vi "Create Measurement Client.vi"() -> ()   [LabVIEW 2021, in "Measurement Client.lvlib"]
uses:
  Measurement Client Utility/Measurement Client.lvlib
  Queue Driver/controls/Queue Operations.ctl
  Measurement Client Utility/subVIs/Data Holder.ctl
  <vilib>/gRPC/LabVIEW gRPC Library/Shared/grpcId.ctl
  <vilib>/Utility/miscctls.llb/LVPoint32TypeDef.ctl
  <vilib>/gRPC/Generated APIs/ni/measurementlink/discovery/v1/RPC Messages/ni_measurementlink_discovery_v1_EnumerateServicesRequest.ctl
  <vilib>/Utility/error.llb/DialogType.ctl
  <vilib>/gRPC/Generated APIs/ni/measurementlink/discovery/v1/ni.measurementlink.discovery.v1.api.lvlib
  <vilib>/Plug-In SDKs/Clients/Discovery V1/NI Discovery V1 Client.lvlib
  <vilib>/gRPC/LabVIEW gRPC Library/grpc-lvsupport-release.lvlib
panel:
  in  "Select All":bool
  in  "Next":bool
  in  "Refresh":bool
  in  "Available Measurements":i32(listbox)
  out "Active Project Name":string
  # "* Project in which the measurement client vi will be created"
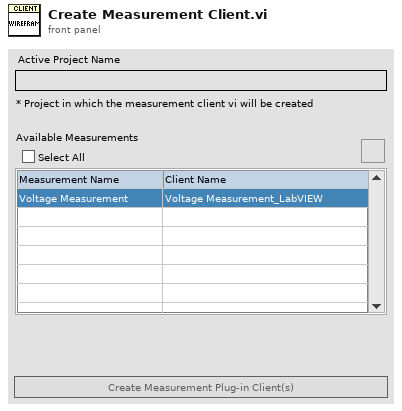
[diagram p1: front panel]
types:
  T1 = typedef "Queue Operations.ctl" = enum16{"Create Q", "Enqueue", "Enqueue N", "Dequeue", "Flush", "Release"}
  T2 = typedef "Measurement Client.lvlib/Data Holder.ctl" = cluster{"gRPCid":T3, "Services":string[][], "MosueDown Coords":T4, "No of Meas":i32, "Select All?":bool}
  T3 = typedef "grpc-lvsupport-release.lvlib/grpcId.ctl" = u64
  T4 = typedef "LVPoint32TypeDef.ctl" = cluster{"Horizontal":i32, "Vertical":i32}
  T5 = enum8{"Enabled", "Disabled", "Disabled and Grayed Out"}
  T6 = typedef "ni.measurementlink.discovery.v1.api.lvlib/ni_measurementlink_discovery_v1_EnumerateServicesRequest.ctl" = cluster{"provided_interface":string}
  T7 = typedef "LVRowAndColumnTypeDef.ctl" = cluster{"Row":i32, "Column":i32}
  T8 = typedef "ni.measurementlink.discovery.v1.api.lvlib/ni_measurementlink_discovery_v1_EnumerateServicesResponse.ctl" = cluster{"available_services":T9[]}
  T9 = typedef "ni.measurementlink.discovery.v1.api.lvlib/ni_measurementlink_discovery_v1_ServiceDescriptor.ctl" = cluster{"display_name":string, "description_url":string, "provided_interfaces":string[], "service_class":string, "annotations":T10[]}
  T10 = typedef "ni.measurementlink.discovery.v1.api.lvlib/ni_measurementlink_discovery_v1_ServiceDescriptor_AnnotationsEntry.ctl" = cluster{"key":string, "value":string}
  T11 = typedef "DialogType.ctl" = u16
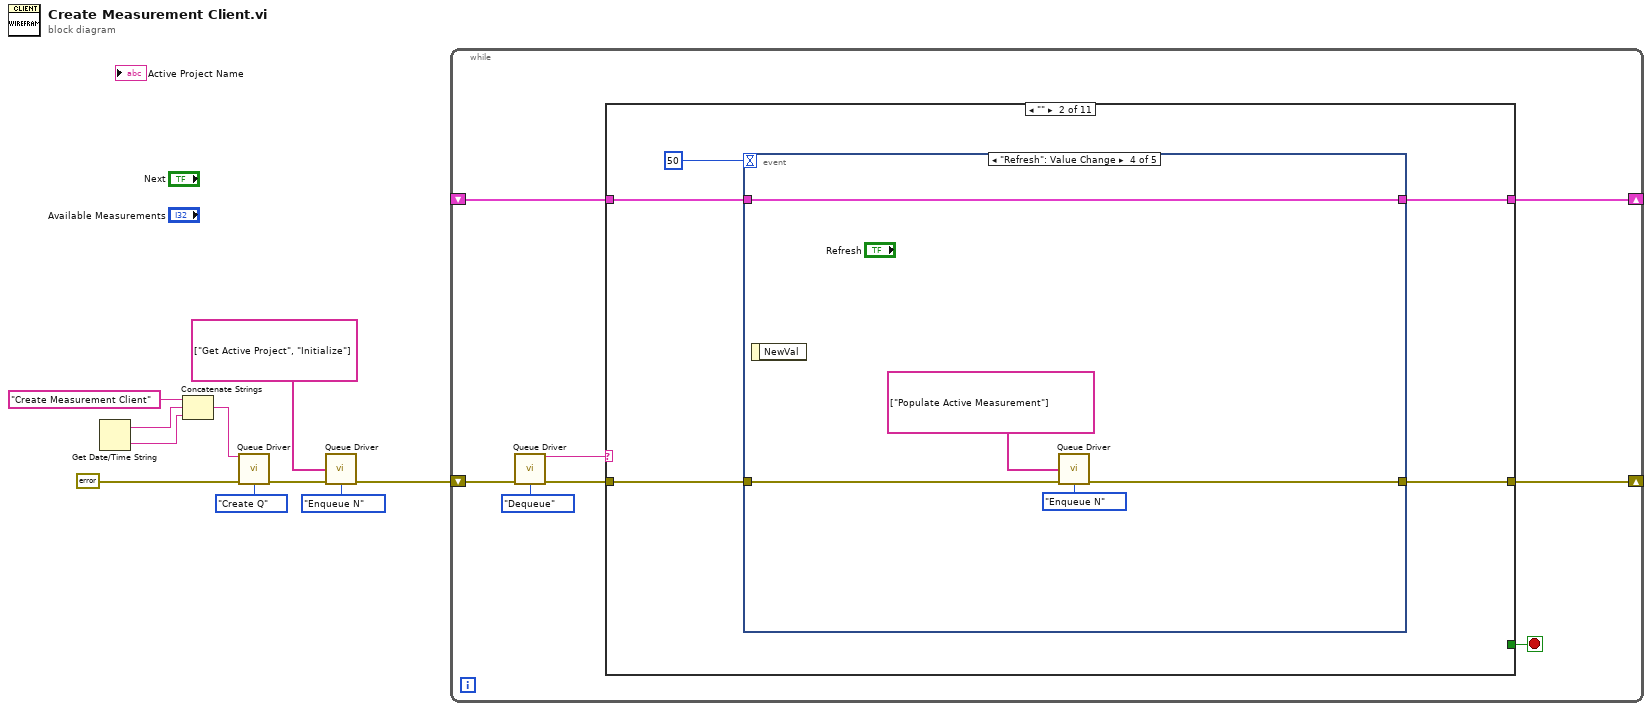
[diagram p0: block diagram]
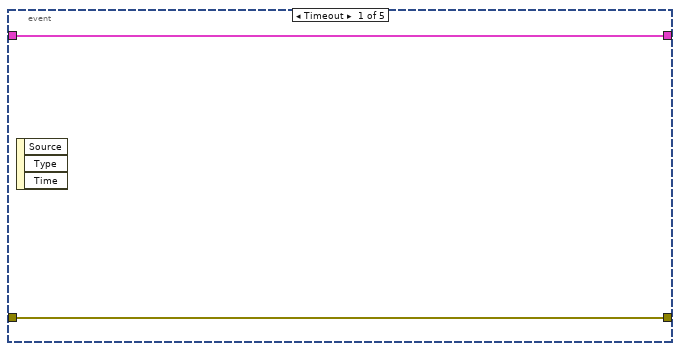
[diagram p3: hidden frame]
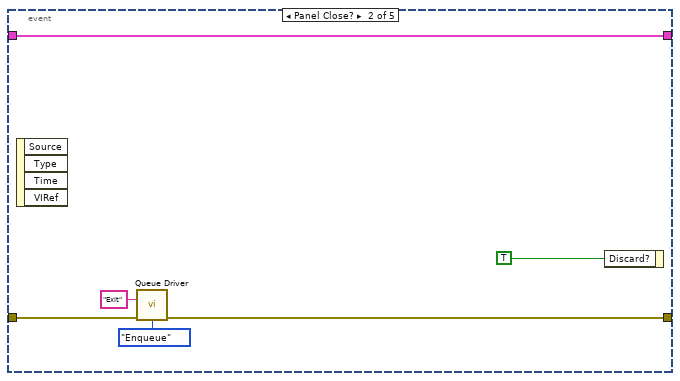
[diagram p4: hidden frame]
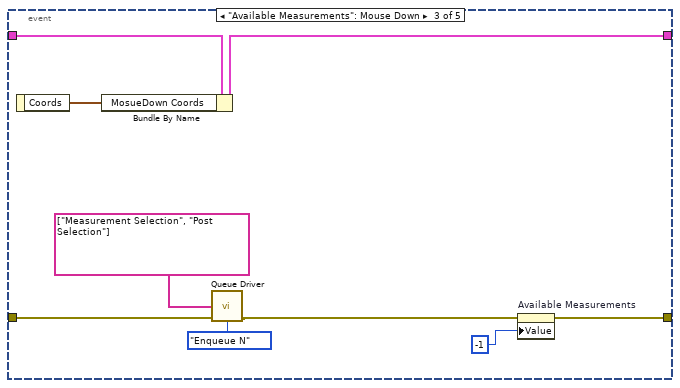
[diagram p5: hidden frame]
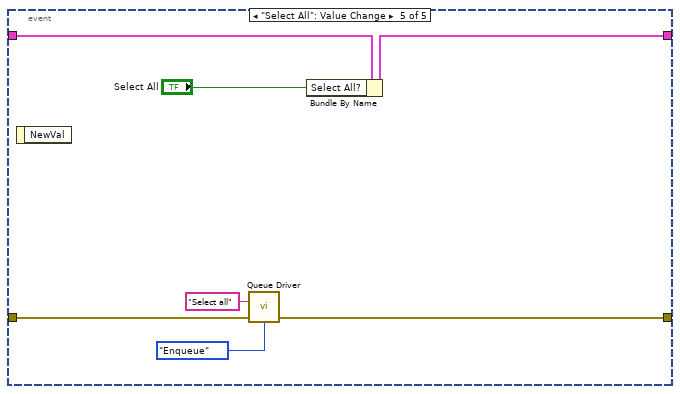
[diagram p6: hidden frame]
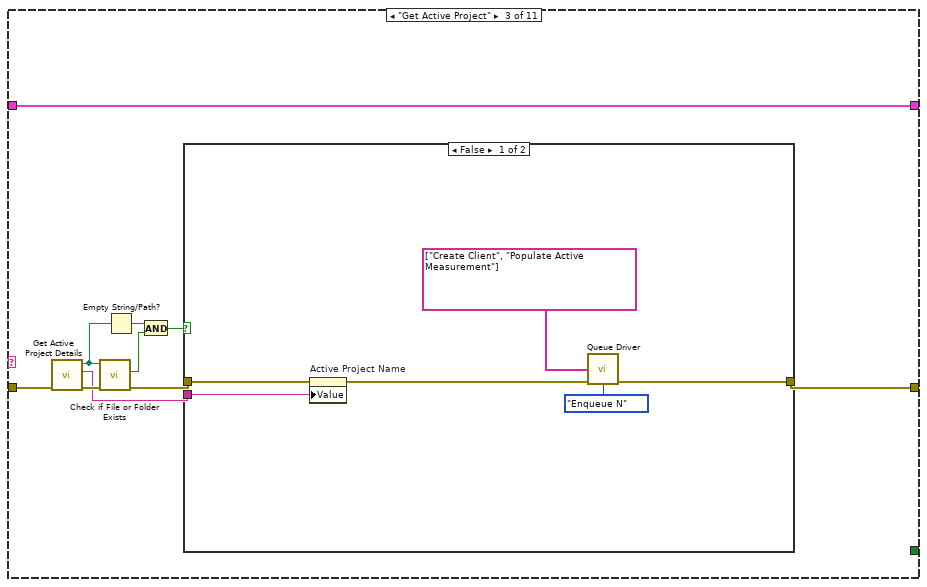
[diagram p7: hidden frame]
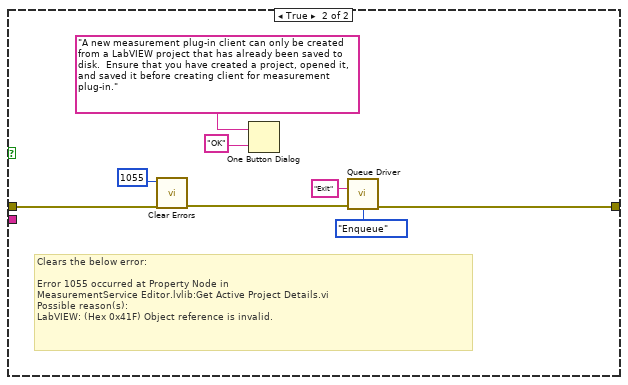
[diagram p8: hidden frame]
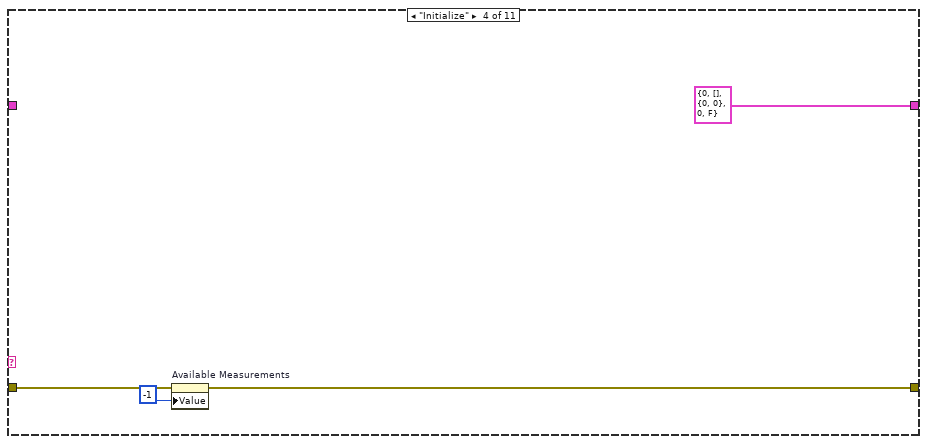
[diagram p9: hidden frame]
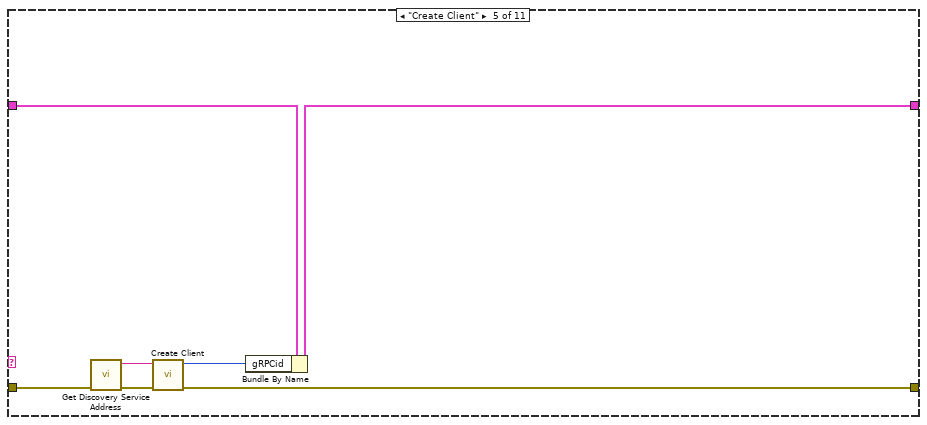
[diagram p10: hidden frame]
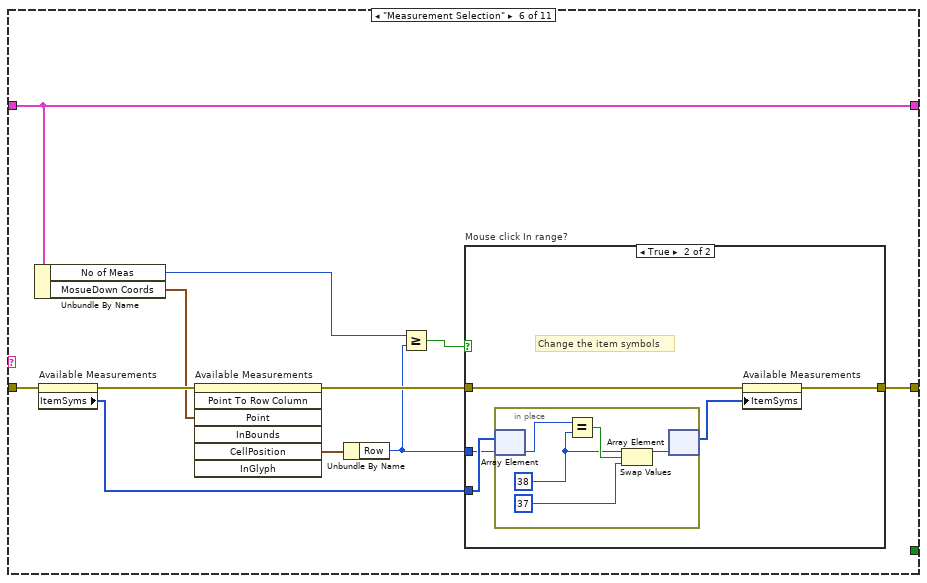
[diagram p11: hidden frame]
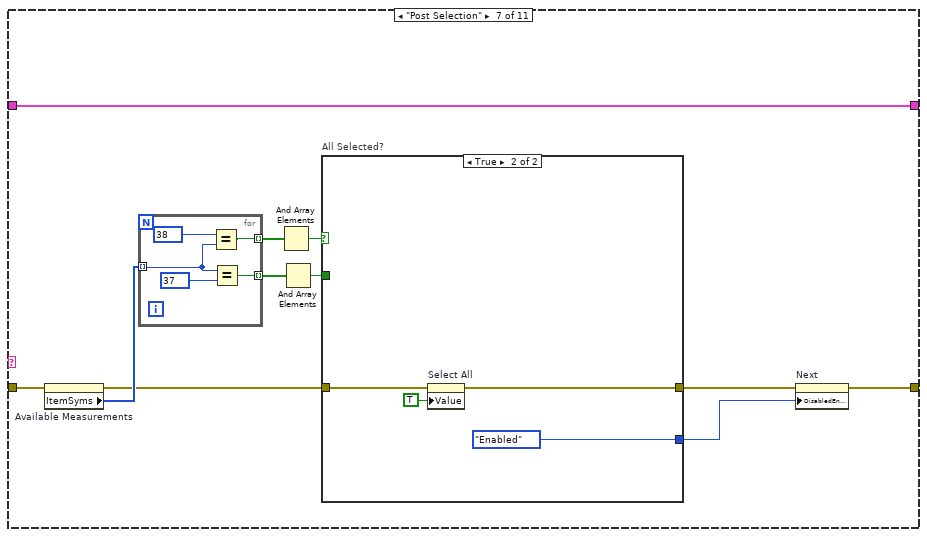
[diagram p13: hidden frame]
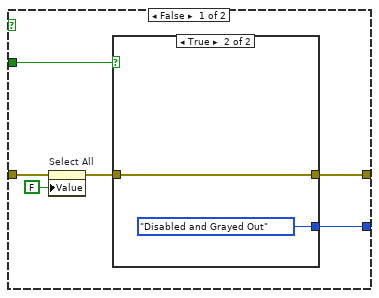
[diagram p14: hidden frame]
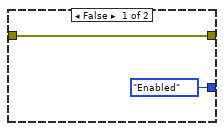
[diagram p15: hidden frame]
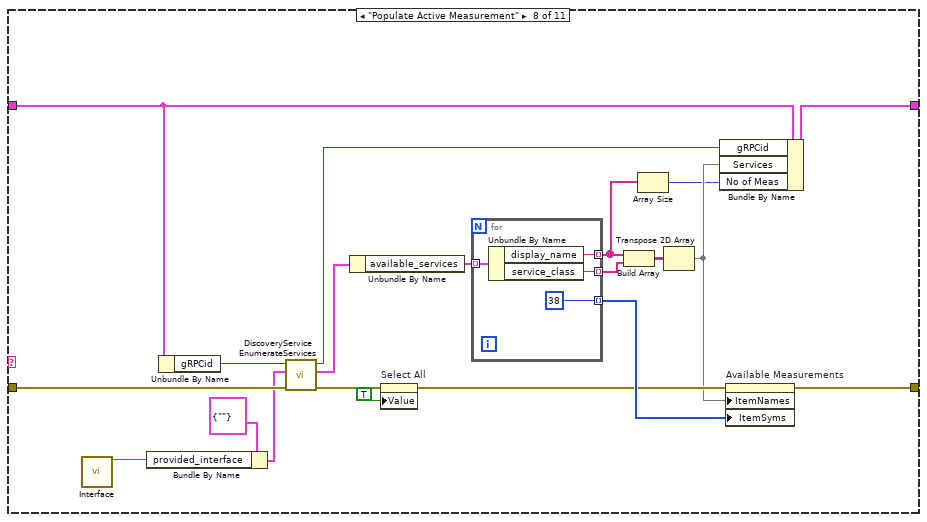
[diagram p16: hidden frame]
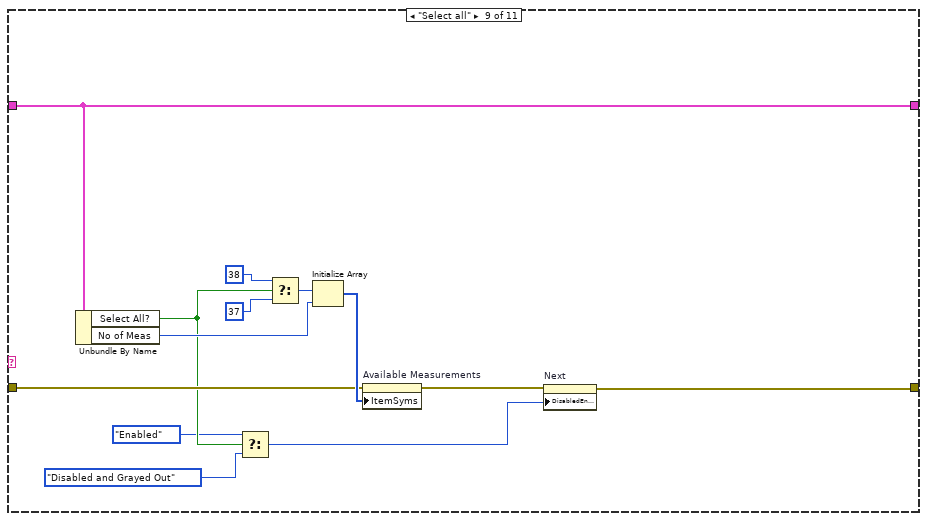
[diagram p17: hidden frame]
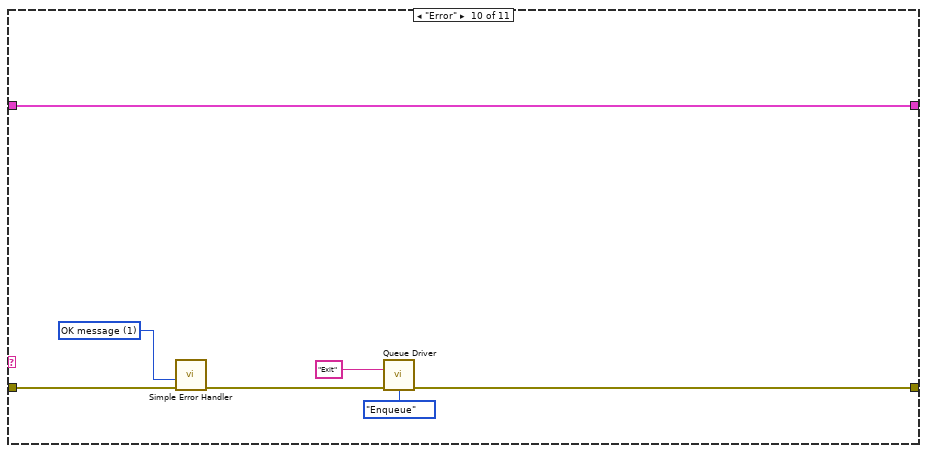
[diagram p18: hidden frame]
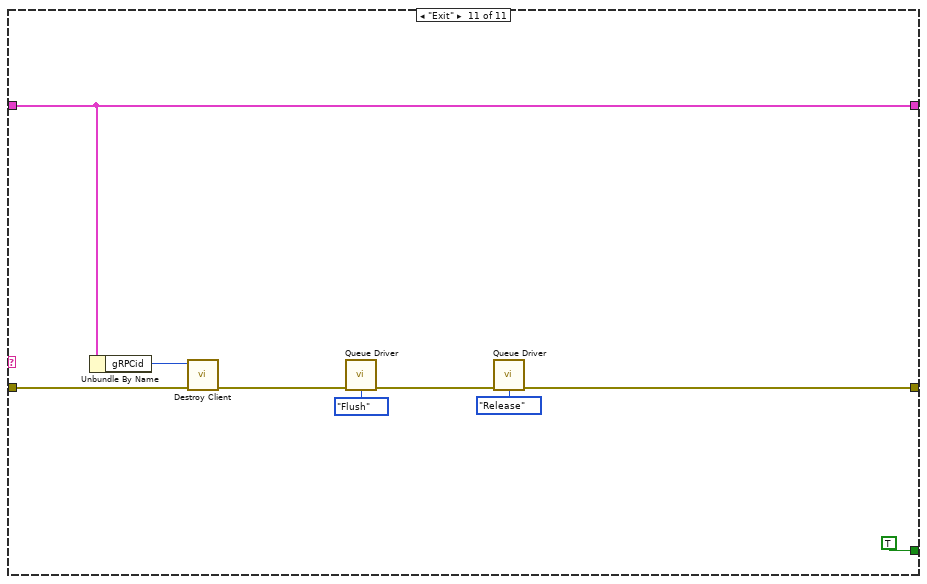
[diagram p19: hidden frame]
diagram:
  n1 = Get Date/Time String() -> (date string=w3:string, time string=w2:string)  [unwired: 3 in]
  n2 = Concatenate Strings("Create Measurement Client" ("Name"), w3, w2) -> (w4:string)
  n3 = call "Queue Driver.vi"("Name"=w4, "error in (no error)"=errorcluster {"status"=FALSE, "code"=0, "source"=""}, "Queue Operations"=Queue_Operations."Create Q") -> ("error out"=w10:errorcluster)  [unwired: 11 in, 1 out]
  n4 = call "Queue Driver.vi"("States[]"=string[] ["Get Active Project", "Initialize"], "error in (no error)"=w10, "Queue Operations"=Queue_Operations."Enqueue N") -> ("error out"=w7:errorcluster)  [unwired: 11 in, 1 out]
  n5 = while {
    shift-right: [w14] -> _
    shift-left: w7 -> [w17]
    shift-right: [w12] -> _
    shift-left: _ -> [w11]
    stop <- w13 stop-if-true
    n6 = call "Queue Driver.vi"("error in (no error)"=w17, "Queue Operations"=Queue_Operations."Dequeue") -> ("Dequeued State"=w15:string, "error out"=w16:errorcluster)  [unwired: 12 in]
    n7 = case shown="\"\"" w15 {
      tunnel: w16 -> [w20 w25 w63 w78 w85 w92 w120 w160 w171 w184 w185]
      tunnel: [w20 w23 w56 w79 w84 w91 w113 w154 w165 w181 w190] -> w14
      tunnel: [_ _ _ _ _ _ _ _ _ _ TRUE] -> w13
      tunnel: [w19 w21 w54 T2 {"gRPCid"=0, "Services"=[], "MosueDown Coords"={"Horizontal"=0, "Vertical"=0}, "No of Meas"=0, "Select All?"=FALSE} ("Data Holder") w83 w93 w121 w153 w177 w178 w188] -> w12
      tunnel: w11 -> [w19 w22 w54 _ w88 w93 w121 w145 w177 w178 w188]
      frame Default {
      }
      frame "" {
        n8 = event shown="[3] \"Refresh\": Value Change" {
          selector: _ -> [_ _ _ _ _]
          dyn-events: _ -> [_ _ _ _ _]
          timeout: 50 -> [_ _ _ _ _]
          tunnel: w25 -> [w27 w31 w35 w44 w53]
          tunnel: [w27 w30 w40 w45 w53] -> w23
          tunnel: w22 -> [w26 w28 w41 w47 w52]
          tunnel: [w26 w28 w39 w47 w51] -> w21
          event Timeout {
            n9 = event-data() -> ()  [unwired: 1 in, 3 out]
          }
          event Panel Close? {
            n10 = event-data() -> ()  [unwired: 1 in, 4 out]
            n11 = call "Queue Driver.vi"("State"="Exit", "error in (no error)"=w31, "Queue Operations"=Queue_Operations."Enqueue") -> ("error out"=w30:errorcluster)  [unwired: 11 in, 1 out]
            n12 = event-data("Discard?"=TRUE) -> ()  [unwired: 1 in, 1 out]
          }
          event "Available Measurements": Mouse Down {
            n13 = event-data() -> ("Coords"=w38:T4)  [unwired: 1 in]
            n14 = Bundle By Name(cluster=w41, "MosueDown Coords"=w38) -> (w39:T2)
            n15 = call "Queue Driver.vi"("States[]"=string[] ["Measurement Selection", "Post Selection"], "error in (no error)"=w35, "Queue Operations"=Queue_Operations."Enqueue N") -> ("error out"=w36:errorcluster)  [unwired: 11 in, 1 out]
            n16 = property on="Available Measurements" class="MCListbox (strict)"(error in=w36, "Value"=-1 ("Available Measurements")) -> (error out=w40:errorcluster)  [unwired: 1 in, 1 out]
          }
          event "Refresh": Value Change {
            n17 = event-data() -> ()  [unwired: 1 in, 1 out]
            n18 = call "Queue Driver.vi"("States[]"=string[] ["Populate Active Measurement"], "error in (no error)"=w44, "Queue Operations"=Queue_Operations."Enqueue N") -> ("error out"=w45:errorcluster)  [unwired: 11 in, 1 out]
          }
          event "Select All": Value Change {
            n19 = event-data() -> ()  [unwired: 1 in, 1 out]
            n20 = call "Queue Driver.vi"("State"="Select all", "Queue Operations"=Queue_Operations."Enqueue") -> ()  [unwired: 12 in, 2 out]
            n21 = Bundle By Name(cluster=w52, "Select All?"="Select All") -> (w51:T2)
          }
        }
      }
      frame "Get Active Project" {
        n22 = call "Get Active Project Details.vi"("error in"=w63) -> ("error out"=w61:errorcluster, "name"=w55:string, "path"=w59:path)  [unwired: 8 in]
        n23 = call <vilib>:"Check if File or Folder Exists.vi"("error in (no error)"=w61, "path"=w59) -> ("error out"=w60:errorcluster, "file or folder exists?"=w57:bool)  [unwired: 7 in, 1 out]
        n24 = Empty String/Path?(string/path=w59) -> (empty?=w62:bool)
        n25 = And(x=w62, y=w57) -> (x .and. y?=w58:bool)
        n26 = case shown="False" w58 {
          tunnel: w60 -> [w68 w75]
          tunnel: [w66 w70] -> w56
          tunnel: w55 -> [w69 _]
          frame False {
            n27 = property on="Active Project Name" class="Str"(error in=w68, "Value"=w69) -> (error out=w65:errorcluster)  [unwired: 1 in, 1 out]
            n28 = call "Queue Driver.vi"("States[]"=string[] ["Create Client", "Populate Active Measurement"], "error in (no error)"=w65, "Queue Operations"=Queue_Operations."Enqueue N") -> ("error out"=w66:errorcluster)  [unwired: 11 in, 1 out]
          }
          frame True {
            # "Clears the below error:\n\nError 1055 occurred at Property Node in \nMeasurementService Editor.lvlib:Get Active Project Details.vi\nPossible reason(s):\nLabVIEW: (Hex 0x41F) Object reference is invalid."
            n29 = call <vilib>:"Clear Errors.vi"("error in (no error)"=w75, "specific error code to clear (0: all)"=1055) -> ("error out"=w74:errorcluster)  [unwired: 4 in, 1 out]
            n30 = One Button Dialog(message="A new measurement plug-in client can only be created from a LabVIEW project that has already been saved to disk.  Ensure that you have created a project, opened it, and saved it before creating client for measurement plug-in.", button name ("OK")="OK") -> ()  [unwired: 1 out]
            n31 = call "Queue Driver.vi"("State"="Exit", "error in (no error)"=w74, "Queue Operations"=Queue_Operations."Enqueue") -> ("error out"=w70:errorcluster)  [unwired: 11 in, 1 out]
          }
        }
      }
      frame "Initialize" {
        n32 = property on="Available Measurements" class="MCListbox (strict)"(error in=w78, "Value"=-1 ("Available Measurements")) -> (error out=w79:errorcluster)  [unwired: 1 in, 1 out]
      }
      frame "Create Client" {
        n33 = call <vilib>:"Get Discovery Service Address.vi"("error in"=w85) -> ("error out"=w86:errorcluster, "address"=w87:string)  [unwired: 9 in]
        n34 = call <vilib>:"Create Client.vi"("error in"=w86, "address"=w87) -> ("error out"=w84:errorcluster, "gRPC ID Out"=w82:T3)  [unwired: 8 in]
        n35 = Bundle By Name(cluster=w88, "gRPCid"=w82) -> (w83:T2)
      }
      frame "Measurement Selection" {
        n36 = Unbundle By Name(w93) -> ("No of Meas"=w99:i32, "MosueDown Coords"=w94:T4)
        n37 = property on="Available Measurements" class="MCListbox (strict)"(error in=w92) -> (error out=w96:errorcluster, "ItemSyms"=w98:i32[])  [unwired: 1 in, 1 out]
        n38 = invoke on="Available Measurements" class="MCListbox (strict)" method="Point To Row Column"(error in=w96, "Point"=w94) -> (error out=w95:errorcluster, "CellPosition"=w90:T7)  [unwired: 5 in, 5 out]
        n39 = Unbundle By Name(w90) -> ("Row"=w89:i32)
        n40 = Greater Or Equal?(x=w99, y=w89) -> (x >= y?=w97:bool)
        n41 = case "Mouse click In range?" shown="True" w97 {
          tunnel: w95 -> [w100 w103]
          tunnel: w98 -> [_ w105]
          tunnel: [w100 w102] -> w91
          tunnel: w89 -> [_ w101]
          frame False {
          }
          frame True {
            # "Change the item symbols"
            n42 = in-place {
              w107 = 38
              n43 = in-place-array #1(w105, w101) -> (w110:i32)
              n44 = Equal?(x=w110, y=w107) -> (x = y?=w109:bool)
              n45 = Swap Values(12:w107, 13:w109, 14:37 ("y")) -> (1:w108:i32)  [unwired: 1 out]
              n46 = in-place-array #1(w108) -> (w104:i32[])  [unwired: 1 out]
            }
            n47 = property on="Available Measurements" class="MCListbox (strict)"(error in=w103, "ItemSyms"=w104) -> (error out=w102:errorcluster)  [unwired: 1 in, 1 out]
          }
        }
      }
      frame "Post Selection" {
        n48 = property on="Available Measurements" class="MCListbox (strict)"(error in=w120) -> (error out=w115:errorcluster, "ItemSyms"=w117:i32[])  [unwired: 1 in, 1 out]
        n49 = for {
          tunnel: w117 -> [w140] mode=indexing
          tunnel: [w139] -> w119 mode=indexing
          tunnel: [w138] -> w118 mode=indexing
          n50 = Equal?(x=38, y=w140) -> (x = y?=w139:bool)
          n51 = Equal?(x=w140, y=37) -> (x = y?=w138:bool)
        }
        n52 = And Array Elements(Boolean array=w119) -> (logical AND=w116:bool)
        n53 = And Array Elements(Boolean array=w118) -> (logical AND=w111:bool)
        n54 = case "All Selected?" shown="True" w116 {
          tunnel: w115 -> [w125 w134]
          tunnel: [w122 w133] -> w114
          tunnel: [w123 T5."Enabled" ("Disabled")] -> w112
          tunnel: w111 -> [w124 _]
          frame False {
            n55 = property on="Select All" class="Bool (strict)"(error in=w125, "Value"=FALSE ("Select All")) -> (error out=w126:errorcluster)  [unwired: 1 in, 1 out]
            n56 = case shown="True" w124 {
              tunnel: w126 -> [w128 w130]
              tunnel: [T5."Enabled" ("Disabled") T5."Disabled and Grayed Out" ("Disabled")] -> w123
              tunnel: [w128 w130] -> w122
              frame False {
              }
              frame True {
              }
            }
          }
          frame True {
            n57 = property on="Select All" class="Bool (strict)"(error in=w134, "Value"=TRUE ("Select All")) -> (error out=w133:errorcluster)  [unwired: 1 in, 1 out]
          }
        }
        n58 = property on="Next" class="Bool"(error in=w114, "DisabledEnum"=w112) -> (error out=w113:errorcluster)  [unwired: 1 in, 1 out]
      }
      frame "Populate Active Measurement" {
        n59 = call "Interface.vi"() -> ("Interface"=w146:string)  [unwired: 15 in]
        n60 = Bundle By Name(cluster=T6 {"provided_interface"=""} ("Request Data"), "provided_interface"=w146) -> (w150:T6)
        n61 = Unbundle By Name(w145) -> ("gRPCid"=w144:T3)
        n62 = call <vilib>:"DiscoveryService EnumerateServices.vi"("error in"=w160, "Request Data"=w150, "gRPC ID"=w144) -> ("error out"=w148:errorcluster, "Response Data"=w159:T8, "gRPC ID out"=w152:T3)  [unwired: 6 in]
        n63 = Unbundle By Name(w159) -> ("available_services"=w158:T9[])
        n64 = property on="Select All" class="Bool (strict)"(error in=w148, "Value"=TRUE ("Select All")) -> (error out=w147:errorcluster)  [unwired: 1 in, 1 out]
        n65 = for {
          tunnel: w158 -> [w164] mode=indexing
          tunnel: [w163] -> w142 mode=indexing
          tunnel: [w162] -> w157 mode=indexing
          tunnel: [38] -> w156 mode=indexing
          n66 = Unbundle By Name(w164) -> ("display_name"=w163:string, "service_class"=w162:string)
        }
        n67 = Build Array(w142, w157) -> (w155:string[][])
        n68 = Array Size(array=w142) -> (size(s)=w141:i32)
        n69 = Transpose 2D Array(2D array=w155) -> (transposed array=w143:string[][])
        n70 = Bundle By Name(cluster=w145, "gRPCid"=w152, "Services"=w143, "No of Meas"=w141) -> (w153:T2)
        n71 = property on="Available Measurements" class="MCListbox (strict)"(error in=w147, "ItemNames"=w143, "ItemSyms"=w156) -> (error out=w154:errorcluster)  [unwired: 1 in, 1 out]
      }
      frame "Select all" {
        n72 = Unbundle By Name(w177) -> ("Select All?"=w169:bool, "No of Meas"=w176:i32)
        n73 = Select(t=T5."Enabled" ("Disabled"), s=w169, f=T5."Disabled and Grayed Out" ("Disabled")) -> (s? t:f=w166:T5)
        n74 = Select(t=38 ("No of Meas"), s=w169, f=37 ("No of Meas")) -> (s? t:f=w173:i32)
        n75 = Initialize Array(w173, w176) -> (w172:i32[])
        n76 = property on="Available Measurements" class="MCListbox (strict)"(error in=w171, "ItemSyms"=w172) -> (error out=w170:errorcluster)  [unwired: 1 in, 1 out]
        n77 = property on="Next" class="Bool"(error in=w170, "DisabledEnum"=w166) -> (error out=w165:errorcluster)  [unwired: 1 in, 1 out]
      }
      frame "Error" {
        w183 = T11 1 items=["no dialog", "OK message", "continue or stop message", "OK message + warnings", "continue/stop + warnings"] ("type of dialog (OK msg:1)")
        n78 = call <vilib>:"Simple Error Handler.vi"("type of dialog (OK msg:1)"=w183, "error in (no error)"=w184) -> ("error out"=w180:errorcluster)  [unwired: 3 in, 4 out]
        n79 = call "Queue Driver.vi"("State"="Exit", "error in (no error)"=w180, "Queue Operations"=Queue_Operations."Enqueue") -> ("error out"=w181:errorcluster)  [unwired: 11 in, 1 out]
      }
      frame "Exit" {
        n80 = Unbundle By Name(w188) -> ("gRPCid"=w187:T3)
        n81 = call <vilib>:"Destroy Client.vi"("error in"=w185, "gRPC ID"=w187) -> ("error out"=w186:errorcluster)  [unwired: 9 in]
        n82 = call "Queue Driver.vi"("error in (no error)"=w186, "Queue Operations"=Queue_Operations."Flush") -> ("error out"=w189:errorcluster)  [unwired: 12 in, 1 out]
        n83 = call "Queue Driver.vi"("error in (no error)"=w189, "Queue Operations"=Queue_Operations."Release") -> ("error out"=w190:errorcluster)  [unwired: 12 in, 1 out]
      }
    }
  }
